vi "Graph InitScale(Mixed).vi"(6 "初回?":bool, 8 "error in (no error)":errorcluster caption="エラー入力（エラーなし）", 9 "ChData":waveform(dbl)[](array[waveform]), 10 "ChName":string[](array[string]), 11 "Mixedグラフ(ref)":refnum<vi>) -> (0 "error out":errorcluster caption="エラー出力", 2 "OK":bool)   [LabVIEW 2014]
panel:
  in  "X軸データ":T1(array[cluster])
  in  "SAVE":bool
  in  "LOAD":bool
  in  "停止":bool
  in  "Y軸データ":T1(array[cluster])
  in  "プロットデータ":T2(array[cluster]) {"MAX" format="%#_6f"; "MIN" format="%#_6f"; "Y軸" items=["No.", "M1回転rpm", "M2回転rpm", "M3回転rpm", "M1トルクN･m", "M2トルクN･m", "M3トルクN･m", ""]}
  # "最大値"
  # "最小値"
  # "Y軸"
  # "表示範囲外！"
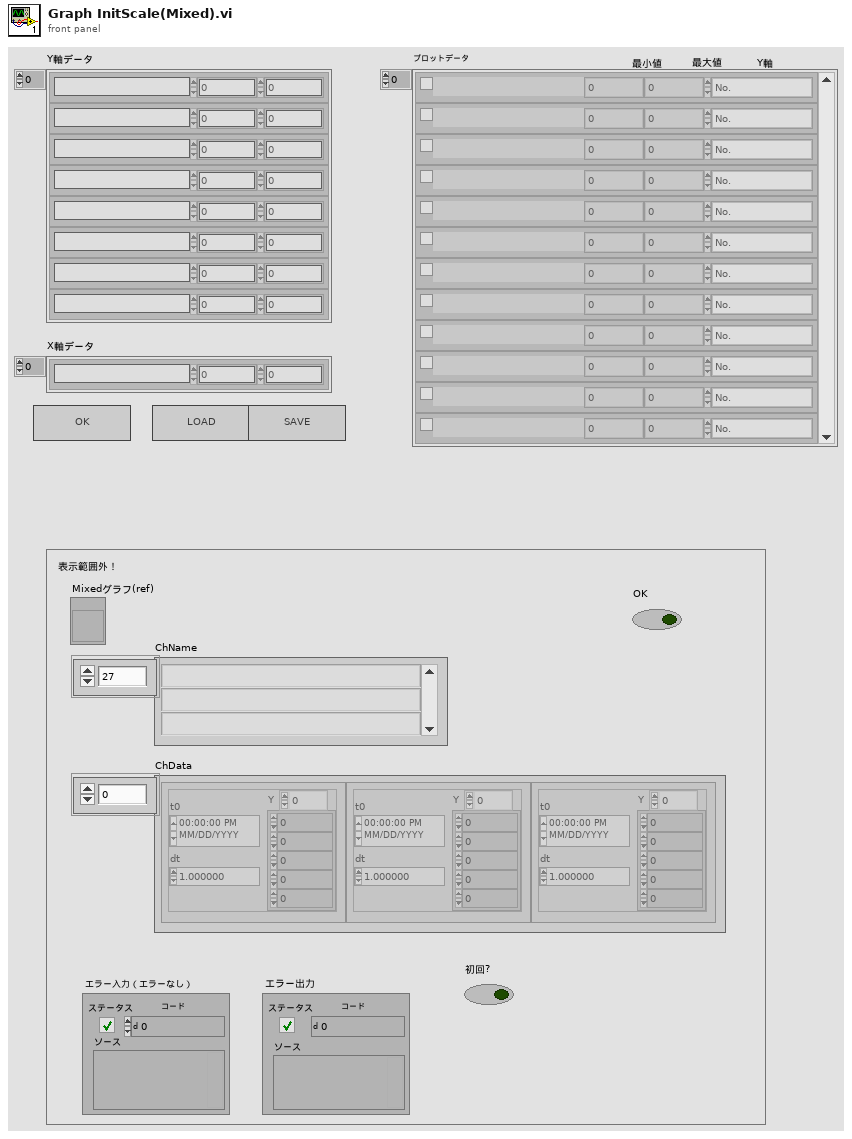
[diagram p1: front panel]
types:
  T1 = cluster{"YLegName":string, "MIN":dbl, "MAX":dbl}[]
  T2 = cluster{"ON/OFF":bool, "CH名称":string, "MIN":dbl, "MAX":dbl, "Y軸":u16}[]
  T3 = enum32{"Invalid", "Standard", "Closed", "Hidden", "Minimized", "Maximized"}
  T4 = cluster{"ON/OFF":bool, "CH名称":string, "MIN":dbl, "MAX":dbl, "Y軸":u16}
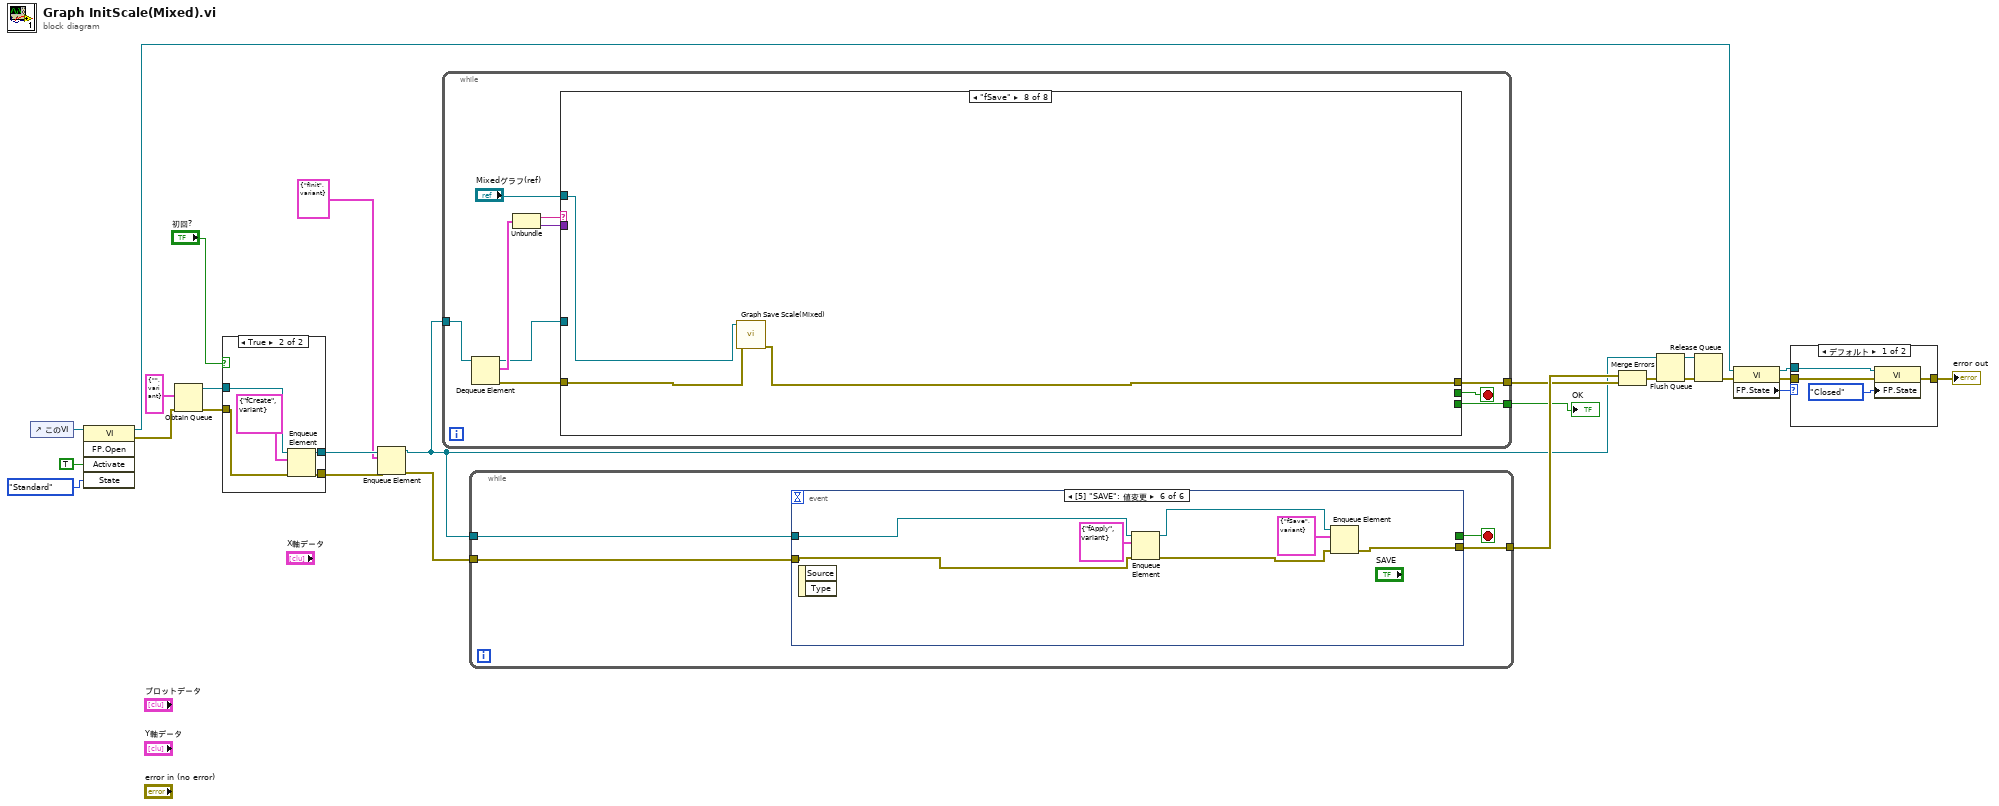
[diagram p0: block diagram]
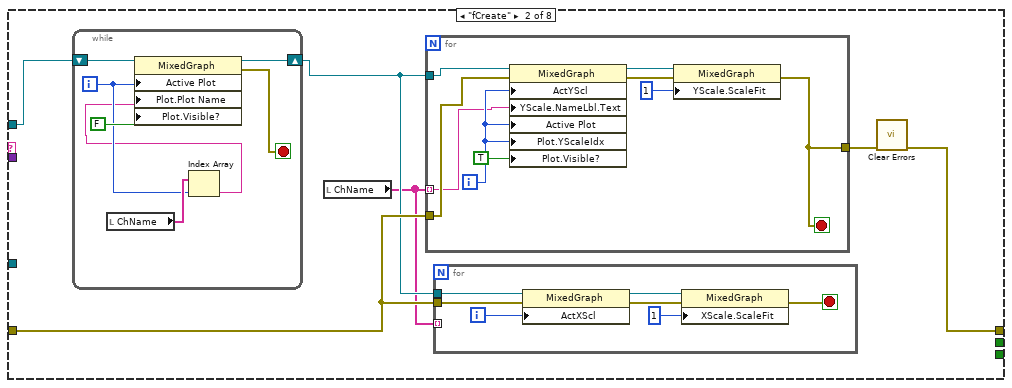
[diagram p5: hidden frame]
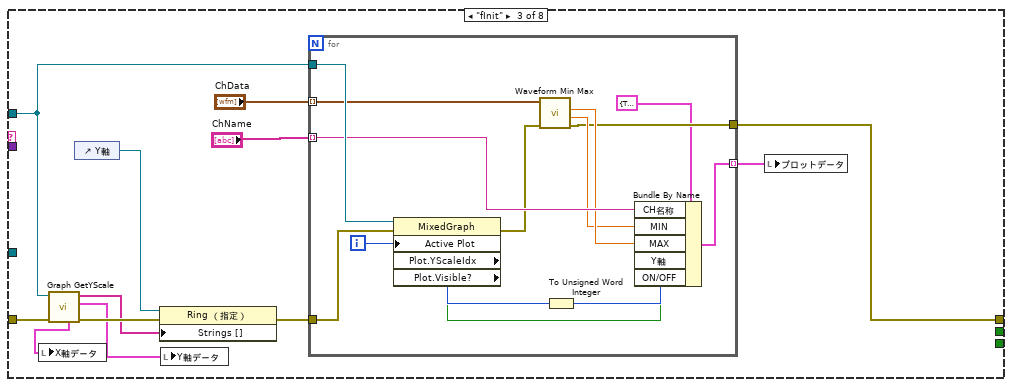
[diagram p6: hidden frame]
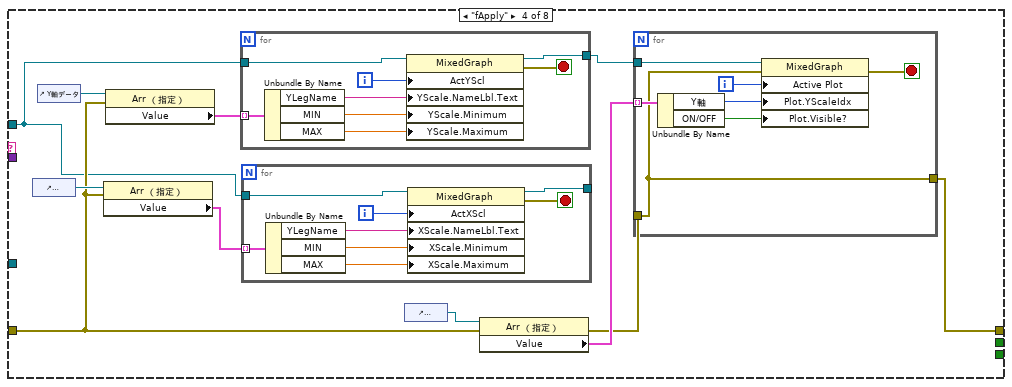
[diagram p7: hidden frame]
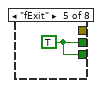
[diagram p8: hidden frame]
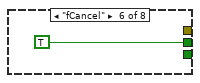
[diagram p9: hidden frame]
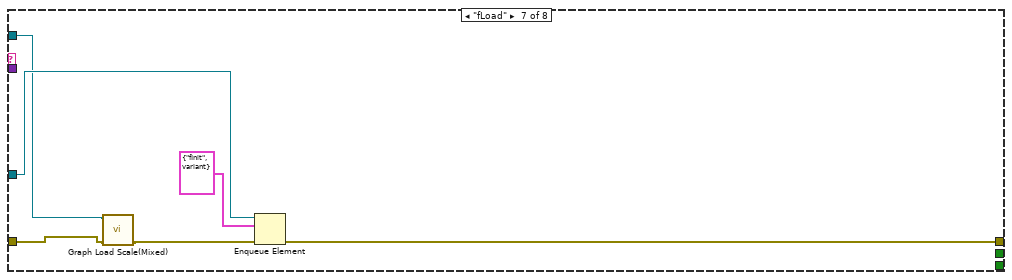
[diagram p10: hidden frame]
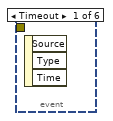
[diagram p11: hidden frame]
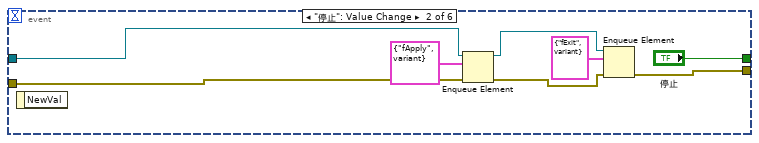
[diagram p12: hidden frame]
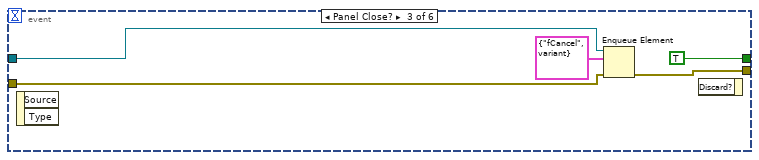
[diagram p13: hidden frame]
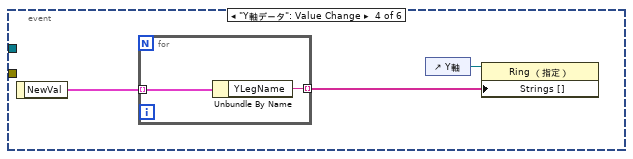
[diagram p14: hidden frame]
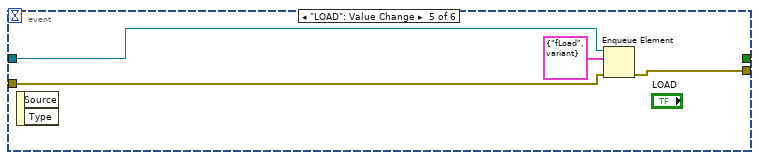
[diagram p15: hidden frame]
diagram:
  n1 = control-ref of="このVI"() -> (w22:refnum<vi>)
  n2 = invoke class="VI" method="FP.Open"(reference=w22, "Activate"=TRUE ("アクティブ化?"), "State"=T3."Standard" ("状態")) -> (reference out=w12:refnum<vi>, error out=w19:errorcluster)  [unwired: 2 in, 3 out]
  n3 = Obtain Queue(element data type=cluster{string, variant} {"", variant}, error in (no error)=w19) -> (queue out=w23:refnum<queue>, error out=w24:errorcluster)  [unwired: 3 in, 1 out]
  n4 = case shown="TRUE" "初回?" {
    tunnel: w24 -> [w27 w32]
    tunnel: [w27 w31] -> w3
    tunnel: w23 -> [w26 w29]
    tunnel: [w26 w28] -> w5
    frame False {
    }
    frame True {
      n5 = Enqueue Element(queue=w29, element=cluster{string, variant} {"fCreate", variant} ("要素"), error in (no error)=w32) -> (queue out=w28:refnum<queue>, error out=w31:errorcluster)  [unwired: 1 in, 1 out]
    }
  }
  n6 = Enqueue Element(queue=w5, element=cluster{string, variant} {"fInit", variant} ("要素"), error in (no error)=w3) -> (queue out=w4:refnum<queue>, error out=w2:errorcluster)  [unwired: 1 in, 1 out]
  n7 = while {
    tunnel: w4 -> [w42]
    tunnel: [w37] -> w17
    tunnel: [w35] -> w13
    stop <- w38 stop-if-true
    n8 = Dequeue Element(queue=w42) -> (queue out=w34:refnum<queue>, element=w41:cluster{string, variant}, error out=w36:errorcluster)  [unwired: 2 in, 1 out]
    n9 = Unbundle(w41) -> (w40:string, w39:variant)
    n10 = case shown="\"fSave\"" w40 {
      tunnel: w39 -> [_ _ _ _ _ _ _ _]
      tunnel: [_ _ _ _ w132 TRUE _ _] -> w38
      tunnel: [_ w48 w75 w102 _ _ w137 w140] -> w37
      tunnel: w36 -> [_ w45 w76 w100 _ _ w136 w141]
      tunnel: "Mixedグラフ(ref)" -> [_ w46 w77 w98 _ _ w134 w142]
      tunnel: [_ _ _ _ w132 _ _ _] -> w35
      tunnel: w34 -> [_ _ _ _ _ _ w138 _]
      frame "FALSE", Default {
      }
      frame "fCreate" {
        n11 = while {
          shift-right: [w61] -> w44
          shift-left: w46 -> [w62]
          i -> [w57]
          stop <- w60 stop-if-true
          n12 = local read "ChName"() -> (w58:string[])
          n13 = Index Array(array=w58, index=w57) -> (element=w56:string)
          n14 = property class="MixedGraph"(reference=w62, "Active Plot"=w57, "Plot.Plot Name"=w56, "Plot.Visible?"=FALSE ("プロット.表示")) -> (reference out=w61:refnum<vi>, error out=w60:errorcluster)  [unwired: 1 in]
        }
        n15 = local read "ChName"() -> (w43:string[])
        n16 = for {
          tunnel: w43 -> [w68] mode=indexing
          tunnel: w44 -> [w71]
          tunnel: w45 -> [w69]
          tunnel: [w63] -> w47
          i -> [w70]
          stop <- w63 stop-if-true
          n17 = property class="MixedGraph"(reference=w71, error in=w69, "ActYScl"=w70, "YScale.NameLbl.Text"=w68, "Active Plot"=w70, "Plot.YScaleIdx"=w70, "Plot.Visible?"=TRUE ("プロット.表示")) -> (reference out=w67:refnum<vi>, error out=w66:errorcluster)
          n18 = property class="MixedGraph"(reference=w67, error in=w66, "YScale.ScaleFit"=u8 1 ("Yスケール.スケールフィット")) -> (error out=w63:errorcluster)  [unwired: 1 out]
        }
        n19 = for {
          tunnel: w45 -> [w50]
          tunnel: w44 -> [w49]
          tunnel: w43 -> [_] mode=indexing
          i -> [w55]
          stop <- w51 stop-if-true
          n20 = property class="MixedGraph"(reference=w49, error in=w50, "ActXScl"=w55) -> (reference out=w54:refnum<vi>, error out=w53:errorcluster)
          n21 = property class="MixedGraph"(reference=w54, error in=w53, "XScale.ScaleFit"=u8 1 ("Yスケール.スケールフィット")) -> (error out=w51:errorcluster)  [unwired: 1 out]
        }
        n22 = call <vilib>:"Clear Errors.vi"("error in (no error)"=w47) -> ("error out"=w48:errorcluster)  [unwired: 5 in, 1 out]
      }
      frame "fInit" {
        n23 = call "Graph GetYScale.vi"("err in"=w76, "GraphChart入力"=w77) -> ("err out"=w82:errorcluster, "Y軸データ"=w78:T1, "Y軸名称"=w81:string[], "X軸データ"=w72:T1)  [unwired: 5 in, 1 out]
        n24 = local write "X軸データ"(w72) -> ()
        n25 = control-ref of="Y軸"() -> (w83:refnum<vi>)
        n26 = property class="Ring （指定）"(reference=w83, error in=w82, "Strings []"=w81) -> (error out=w80:errorcluster)  [unwired: 1 out]
        n27 = local write "Y軸データ"(w78) -> ()
        n28 = for {
          tunnel: "ChName" -> [w93] mode=indexing
          tunnel: w77 -> [w97]
          tunnel: "ChData" -> [w95] mode=indexing
          tunnel: w80 -> [w94]
          tunnel: [w88] -> w79 mode=indexing
          tunnel: [w86] -> w75
          i -> [w96]
          n29 = property class="MixedGraph"(reference=w97, error in=w94, "Active Plot"=w96) -> (error out=w87:errorcluster, "Plot.YScaleIdx"=w90:u32, "Plot.Visible?"=w84:bool)  [unwired: 1 out]
          n30 = call <vilib>:"Waveform Min Max.vi"("error in (no error)"=w87, "waveform in"=w95) -> ("error out"=w86:errorcluster, "Y min"=w91:dbl, "Y max"=w92:dbl)  [unwired: 4 in, 3 out]
          n31 = To Unsigned Word Integer(number=w90) -> (unsigned 16bit integer=w89:u16)
          n32 = Bundle By Name(cluster=T4 {"ON/OFF"=TRUE, "CH名称"="", "MIN"=0.0, "MAX"=0.0, "Y軸"=0} ("クラスタ"), "CH名称"=w93, "MIN"=w91, "MAX"=w92, "Y軸"=w89, "ON/OFF"=w84) -> (w88:T4)
        }
        n33 = local write "プロットデータ"(w79) -> ()
      }
      frame "fApply" {
        n34 = control-ref of="X軸データ"() -> (w101:refnum<vi>)
        n35 = control-ref of="Y軸データ"() -> (w108:refnum<vi>)
        n36 = property class="Arr （指定）"(reference=w101, error in=w100) -> ("Value"=w99:T1)  [unwired: 2 out]
        n37 = property class="Arr （指定）"(reference=w108, error in=w100) -> ("Value"=w107:T1)  [unwired: 2 out]
        n38 = for {
          tunnel: w98 -> [w131]
          tunnel: w107 -> [w129] mode=indexing
          tunnel: [w124] -> w104
          i -> [w130]
          stop <- w125 stop-if-true
          n39 = Unbundle By Name(w129) -> ("YLegName"=w128:string, "MIN"=w127:dbl, "MAX"=w126:dbl)
          n40 = property class="MixedGraph"(reference=w131, "ActYScl"=w130, "YScale.NameLbl.Text"=w128, "YScale.Minimum"=w127, "YScale.Maximum"=w126) -> (reference out=w124:refnum<vi>, error out=w125:errorcluster)  [unwired: 1 in]
        }
        n41 = for {
          tunnel: w98 -> [w116]
          tunnel: w99 -> [w114] mode=indexing
          tunnel: [w109] -> _
          i -> [w115]
          stop <- w110 stop-if-true
          n42 = Unbundle By Name(w114) -> ("YLegName"=w113:string, "MIN"=w112:dbl, "MAX"=w111:dbl)
          n43 = property class="MixedGraph"(reference=w116, "ActXScl"=w115, "XScale.NameLbl.Text"=w113, "XScale.Minimum"=w112, "XScale.Maximum"=w111) -> (reference out=w109:refnum<vi>, error out=w110:errorcluster)  [unwired: 1 in]
        }
        n44 = control-ref of="プロットデータ"() -> (w106:refnum<vi>)
        n45 = property class="Arr （指定）"(reference=w106, error in=w100) -> (error out=w103:errorcluster, "Value"=w105:T2)  [unwired: 1 out]
        n46 = for {
          tunnel: w105 -> [w123] mode=indexing
          tunnel: w104 -> [w122]
          tunnel: w103 -> [w118]
          tunnel: [w118] -> w102
          i -> [w121]
          stop <- w119 stop-if-true
          n47 = Unbundle By Name(w123) -> ("Y軸"=w120:u16, "ON/OFF"=w117:bool)
          n48 = property class="MixedGraph"(reference=w122, error in=w118, "Active Plot"=w121, "Plot.YScaleIdx"=w120, "Plot.Visible?"=w117) -> (error out=w119:errorcluster)  [unwired: 1 out]
        }
      }
      frame "fExit" {
        w132 = TRUE
      }
      frame "fCancel" {
      }
      frame "fLoad" {
        n49 = call "Graph Load Scale(Mixed).vi"("err in"=w136, "MixedGraph入力"=w134) -> ("err out"=w135:errorcluster)  [unwired: 9 in]
        n50 = Enqueue Element(queue=w138, element=cluster{string, variant} {"fInit", variant} ("要素"), error in (no error)=w135) -> (error out=w137:errorcluster)  [unwired: 1 in, 2 out]
      }
      frame "fSave" {
        n51 = call "Graph Save Scale(Mixed).vi"("err in"=w141, "MixedGraph入力"=w142) -> ("error out"=w140:errorcluster)  [unwired: 9 in]
      }
    }
  }
  "OK" <- w13
  n52 = while {
    tunnel: w4 -> [w145]
    tunnel: w2 -> [w144]
    tunnel: [w143] -> w18
    stop <- w146 stop-if-true
    n53 = event shown="[5] \"SAVE\": 値変更" {
      selector: _ -> [_ _ _ _ _ _]
      dyn-events: _ -> [_ _ _ _ _ _]
      timeout: _ -> [_ _ _ _ _ _]
      tunnel: [_ "停止" TRUE ("停止") _ _ _] -> w146
      tunnel: w145 -> [_ w148 w157 _ w167 w169]
      tunnel: w144 -> [_ w149 w156 _ w166 w172]
      tunnel: [_ w152 w155 _ w165 w174] -> w143
      event Timeout {
        n54 = event-data() -> ()  [unwired: 1 in, 3 out]
      }
      event "停止": Value Change {
        n55 = event-data() -> ()  [unwired: 1 in, 1 out]
        n56 = Enqueue Element(queue=w148, element=cluster{string, variant} {"fApply", variant} ("要素"), error in (no error)=w149) -> (queue out=w147:refnum<queue>, error out=w150:errorcluster)  [unwired: 1 in, 1 out]
        n57 = Enqueue Element(queue=w147, element=cluster{string, variant} {"fExit", variant} ("要素"), error in (no error)=w150) -> (error out=w152:errorcluster)  [unwired: 1 in, 2 out]
      }
      event Panel Close? {
        n58 = event-data() -> ()  [unwired: 1 in, 2 out]
        n59 = Enqueue Element(queue=w157, element=cluster{string, variant} {"fCancel", variant} ("要素"), error in (no error)=w156) -> (error out=w155:errorcluster)  [unwired: 1 in, 2 out]
        n60 = event-data() -> ()  [unwired: 2 in, 1 out]
      }
      event "Y軸データ": Value Change {
        n61 = event-data() -> ("NewVal"=w162:T1)  [unwired: 1 in]
        n62 = for {
          tunnel: w162 -> [w164] mode=indexing
          tunnel: [w163] -> w160 mode=indexing
          n63 = Unbundle By Name(w164) -> ("YLegName"=w163:string)
        }
        n64 = control-ref of="Y軸"() -> (w161:refnum<vi>)
        n65 = property class="Ring （指定）"(reference=w161, "Strings []"=w160) -> ()  [unwired: 1 in, 2 out]
      }
      event "LOAD": Value Change {
        n66 = event-data() -> ()  [unwired: 1 in, 2 out]
        n67 = Enqueue Element(queue=w167, element=cluster{string, variant} {"fLoad", variant} ("要素"), error in (no error)=w166) -> (error out=w165:errorcluster)  [unwired: 1 in, 2 out]
      }
      event "SAVE": Value Change {
        n68 = event-data() -> ()  [unwired: 1 in, 2 out]
        n69 = Enqueue Element(queue=w169, element=cluster{string, variant} {"fApply", variant} ("要素"), error in (no error)=w172) -> (queue out=w170:refnum<queue>, error out=w171:errorcluster)  [unwired: 1 in, 1 out]
        n70 = Enqueue Element(queue=w170, element=cluster{string, variant} {"fSave", variant} ("要素"), error in (no error)=w171) -> (error out=w174:errorcluster)  [unwired: 1 in, 2 out]
      }
    }
  }
  n71 = Merge Errors(w18, w17) -> (w16:errorcluster)
  n72 = Flush Queue(queue=w4, error in (no error)=w16) -> (queue out=w14:refnum<queue>, error out=w15:errorcluster)  [unwired: 1 out]
  n73 = Release Queue(queue=w14, error in (no error)=w15) -> (error out=w11:errorcluster)  [unwired: 1 in, 2 out]
  n74 = property class="VI"(reference=w12, error in=w11) -> (reference out=w9:refnum<vi>, error out=w8:errorcluster, "FP.State"=w10:T3)
  n75 = case shown="デフォルト" w10 {
    tunnel: w9 -> [w178 _]
    tunnel: w8 -> [w177 w180]
    tunnel: [w176 w180] -> w7
    frame Default {
      n76 = property class="VI"(reference=w178, error in=w177, "FP.State"=T3."Closed" ("フロントパネルウィンドウ:状態")) -> (error out=w176:errorcluster)  [unwired: 1 out]
    }
    frame "Invalid", "Closed" {
    }
  }
  "error out" <- w7
